vi "Read All Image Pixels.vi"(0 "fpga inteface in":refnum<k20>, 5 "display channel number":i32, 7 "image bytes":u32, 11 "error in (no error)":errorcluster) -> (4 "fpga interface out":refnum<k20>, 6 "image pixel data region":refnum<data-value>, 8 "elements in region":u32, 15 "error out":errorcluster)   [LabVIEW 2023, in "GettingStarted_Common_148X_Host.lvlib"]
uses:
  GettingStarted_Common_148X_Host.lvlib
  <instrlib>/_niInstr/Data Manipulation/v1/Host/niInstr Data Manipulation v1 Host.lvlib
  <instrlib>/_niInstr/Data Manipulation/v1/Host/Private/Copy to New External Data Value Reference U81D.vi
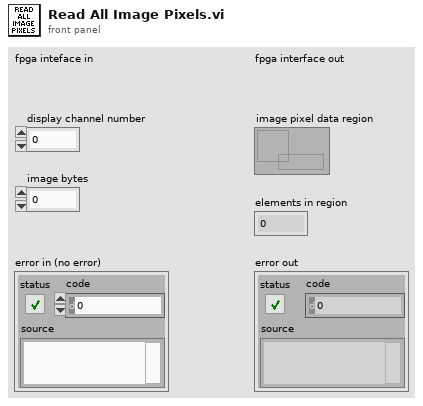
[diagram p1: front panel]
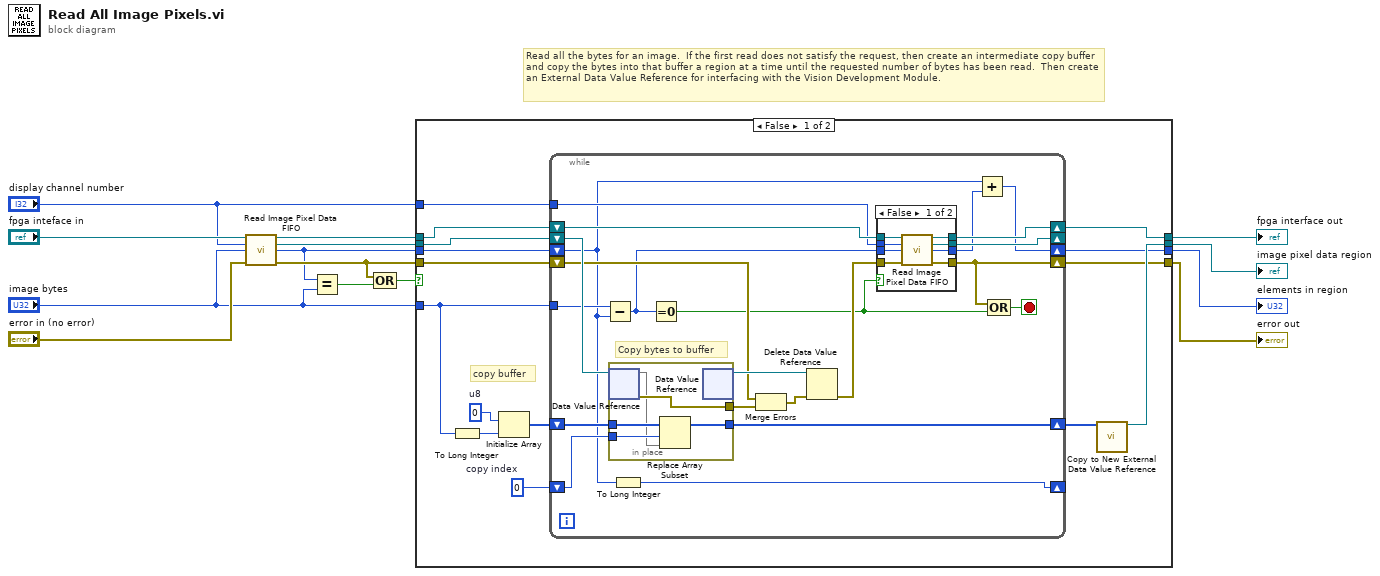
[diagram p0: block diagram]
diagram:
  # "Read all the bytes for an image.  If the first read does not satisfy the request, then create an intermediate copy buffer and copy the bytes into that buffer a region at a time until the requested number of bytes has been read.  Then create an External Data Value Reference for interfacing with the Vision Development Module."
  n1 = call "Read Image Pixel Data FIFO.vi"("fpga inteface in"="fpga inteface in", "display channel number"="display channel number", "number of elements"="image bytes", "error in (no error)"="error in (no error)") -> ("fpga interface out"=w12:refnum<k20>, "image pixel data region"=w8:refnum<data-value>, "elements in region"=w2:u32, "error out"=w9:errorcluster)  [unwired: 7 in, 1 out]
  n2 = Equal?(x=w2, y="image bytes") -> (x = y?=w4:bool)
  n3 = Compound Arithmetic op=OR(w9, w4) -> (w10:bool)
  n4 = case shown="False" w10 {
    tunnel: w12 -> [w19 w70]
    tunnel: [w18 w70] -> w11
    tunnel: w9 -> [w25 w68]
    tunnel: w8 -> [w27 w69]
    tunnel: [w23 w69] -> w6
    tunnel: [w22 w68] -> w7
    tunnel: w2 -> [w21 w67]
    tunnel: [w16 w67] -> w5
    tunnel: "image bytes" -> [w20 _]
    tunnel: "display channel number" -> [w17 _]
    frame False {
      w15 = 0  # copy index
      w29 = u8 0  # u8
      # "copy buffer"
      n5 = To Long Integer(number=w20) -> (32bit integer=w28:i32)
      n6 = Initialize Array(w29, w28) -> (w26:u8[])
      n7 = while {
        shift-right: [w45] -> w24
        shift-left: w26 -> [w50]
        shift-right: [w30] -> w22
        shift-left: w25 -> [w47]
        tunnel: w20 -> [w44]
        shift-right: [w41] -> w18
        shift-left: w19 -> [w43]
        shift-right: [w40] -> _
        shift-left: w27 -> [w51]
        shift-right: [w37] -> w16
        shift-left: w21 -> [w34]
        tunnel: w17 -> [w39]
        shift-right: [w33] -> _
        shift-left: w15 -> [w35]
        stop <- w32 stop-if-true
        # "Copy bytes to buffer"
        n8 = Subtract(x=w44, y=w34) -> (x-y=w36:u32)
        n9 = in-place {
          in-place-border: w50 -> [w56]
          in-place-border: [w55] -> w45
          in-place-border: [w54] -> w48
          in-place-border: w35 -> [w53]
          n10 = in-place-dvr #1(w51) -> (w52:u8[], w54:errorcluster)
          n11 = Replace Array Subset(array=w56, new element=w52, index=w53) -> (w55:u8[])
          n12 = in-place-dvr #1() -> (w49:refnum<data-value>)  [unwired: 1 in, 1 out]
        }
        n13 = To Long Integer(number=w34) -> (32bit integer=w33:i32)
        n14 = Equal To 0?(x=w36) -> (x = 0?=w31:bool)
        n15 = Merge Errors(w47, w48) -> (w46:errorcluster)
        n16 = Delete Data Value Reference(data value reference=w49, error in=w46) -> (error out=w42:errorcluster)  [unwired: 1 out]
        n17 = case shown="False" w31 {
          tunnel: w43 -> [w64 w66]
          tunnel: w42 -> [w63 w65]
          tunnel: [w62 w65] -> w30
          tunnel: [w61 w66] -> w41
          tunnel: [w60 _] -> w40
          tunnel: w39 -> [w59 _]
          tunnel: [w58 _] -> w38
          tunnel: w36 -> [w57 _]
          frame False {
            n18 = call "Read Image Pixel Data FIFO.vi"("fpga inteface in"=w64, "display channel number"=w59, "number of elements"=w57, "error in (no error)"=w63) -> ("fpga interface out"=w61:refnum<k20>, "image pixel data region"=w60:refnum<data-value>, "elements in region"=w58:u32, "error out"=w62:errorcluster)  [unwired: 7 in, 1 out]
          }
          frame True {
          }
        }
        n19 = Add(x=w34, y=w38) -> (x+y=w37:u32)
        n20 = Compound Arithmetic op=OR(w30, w31) -> (w32:bool)
      }
      n21 = call-poly <instrlib>:"Copy to New External Data Value Reference.vi"("array"=w24) -> ("output array reference"=w23:refnum<data-value>)  [unwired: 13 in, 1 out]
    }
    frame True {
    }
  }
  "fpga interface out" <- w11
  "error out" <- w7
  "image pixel data region" <- w6
  "elements in region" <- w5
